vi "Step.vi"(8 "error in":errorcluster, 11 "class data in":refnum<class "Ball.lvclass">) -> (0 "error out":errorcluster, 3 "class data out":refnum<class "Ball.lvclass">)   [LabVIEW 2010, in "Labricks.lvlib" / "Ball.lvclass"]
uses:
  Ball.lvclass
  Ball.lvclass/Ball.ctl
  RenderBase/SceneObject_class/properties/Position/GetPosition.vi
  RenderBase/Sprite_class/properties/Direction/GetDirection.vi
  RenderBase/SceneObject_class/SceneObject.lvclass
  RenderBase/Sprite_class/Sprite.lvclass
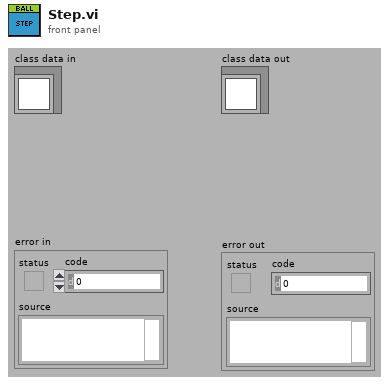
[diagram p1: front panel]
types:
  T1 = typedef "LV3DPointTypeDef.ctl" = cluster{"X":sgl, "Y":sgl, "Z":sgl}
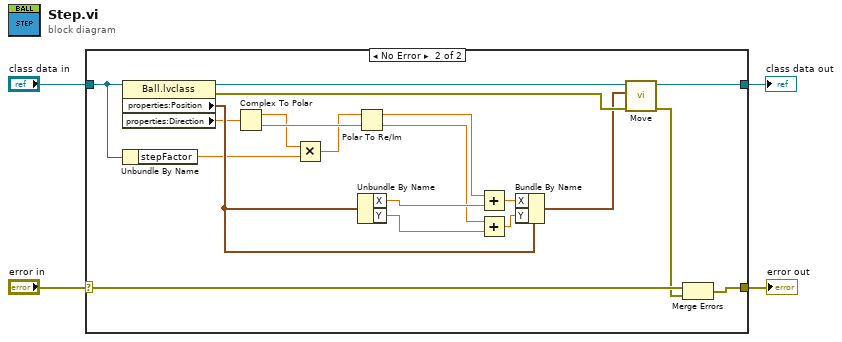
[diagram p0: block diagram]
diagram:
  n1 = case shown="No Error" "error in" {
    selector: "error in" -> [w5 w21]
    tunnel: [w6 w24] -> w4
    tunnel: "class data in" -> [w6 w8]
    tunnel: [w5 w20] -> w1
    frame Error {
    }
    frame No Error {
      n2 = property class="Ball.lvclass"(reference=w8) -> (reference out=w26:refnum<class "Ball.lvclass">, error out=w23:errorcluster, "properties:Position"=w25:T1, "properties:Direction"=w14:csg)  [unwired: 1 in]
      n3 = Unbundle By Name(w8) -> ("stepFactor"=w7:sgl)
      n4 = Complex To Polar(r * e^(i*theta)=w14) -> (r=w12:sgl, theta=w13:sgl)
      n5 = Multiply(x=w12, y=w7) -> (x*y=w11:sgl)
      n6 = Polar To Re/Im(2:w13, 3:w11) -> (0:w9:sgl, 1:w10:sgl)
      n7 = Unbundle By Name(w25) -> ("X"=w15:sgl, "Y"=w17:sgl)
      n8 = Add(x=w10, y=w15) -> (x+y=w16:sgl)
      n9 = Add(x=w9, y=w17) -> (x+y=w18:sgl)
      n10 = Bundle By Name(cluster=w25, "X"=w16, "Y"=w18) -> (w22:T1)
      n11 = call-dynamic "Move.vi"("error in (no error)"=w23, "targetCoords in"=w22, "class data in"=w26) -> ("error out"=w19:errorcluster, "class data out"=w24:refnum<class "Ball.lvclass">)  [unwired: 7 in]
      n12 = Merge Errors(w21, w19) -> (w20:errorcluster)
    }
  }
  "error out" <- w1
  "class data out" <- w4
